vi "mainvi.vi"() -> ()   [LabVIEW 2013]
uses:
  class2/class2.lvclass
  mainclass/mainclass.lvclass
panel:
  out "now place 4":cluster{"x":dbl, "y":dbl}
  in  "stop":bool
  out "now place 3":cluster{"x":dbl, "y":dbl}
  out "now place 2":cluster{"x":dbl, "y":dbl}
  in  "now place":cluster{"x":dbl, "y":dbl}
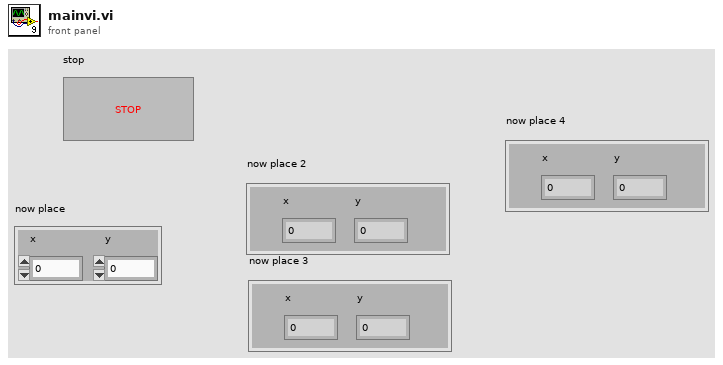
[diagram p1: front panel]
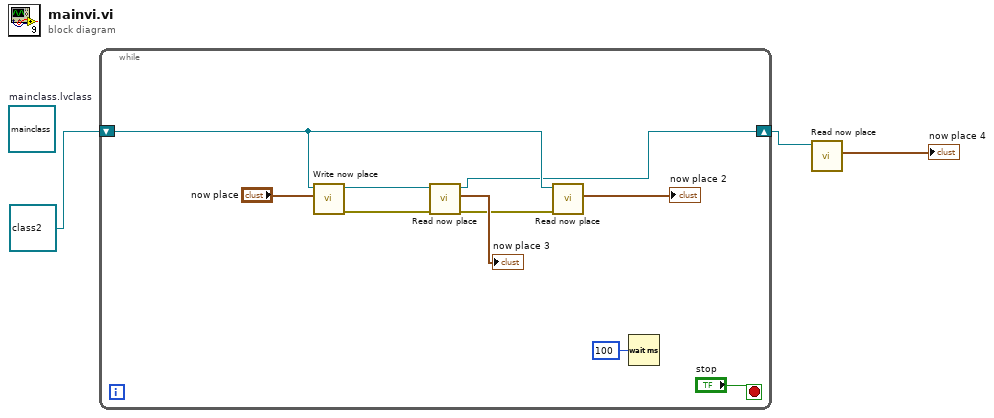
[diagram p0: block diagram]
diagram:
  (unwired) refnum<class "mainclass.lvclass"> refnum  # mainclass.lvclass
  n1 = while {
    shift-right: [w4] -> w2
    shift-left: refnum<class "class2.lvclass"> refnum ("class2.lvclass") -> [w5]
    stop <- "stop" stop-if-true
    n2 = call-dynamic "Write now place.vi"("now place"="now place", "mainclass in"=w5) -> ("error out"=w9:errorcluster, "mainclass out"=w11:refnum<class "class2.lvclass">)  [unwired: 8 in]
    n3 = call-dynamic "Read now place.vi"("error in (no error)"=w9, "mainclass in"=w11) -> ("error out"=w8:errorcluster, "now place"=→"now place 3":cluster{"x":dbl, "y":dbl}, "mainclass out"=w4:refnum<class "class2.lvclass">)  [unwired: 7 in]
    n4 = call-dynamic "Read now place.vi"("error in (no error)"=w8, "mainclass in"=w5) -> ("now place"=→"now place 2":cluster{"x":dbl, "y":dbl})  [unwired: 7 in, 2 out]
    n5 = Wait (ms)(milliseconds to wait=u32 100) -> ()  [unwired: 1 out]
  }
  n6 = call-dynamic "Read now place.vi"("mainclass in"=w2) -> ("now place"=→"now place 4":cluster{"x":dbl, "y":dbl})  [unwired: 8 in, 2 out]
